vi "_29_Sample_qsns_9[5].vi"() -> ()   [LabVIEW 2020]
panel:
  out "subarray 3":i32[](array[numeric])
  out "subarray 2":i32[](array[numeric])
  out "subarray":i32[](array[numeric])
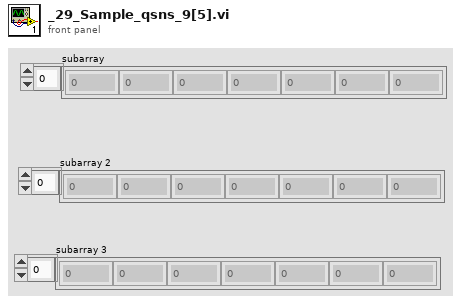
[diagram p1: front panel]
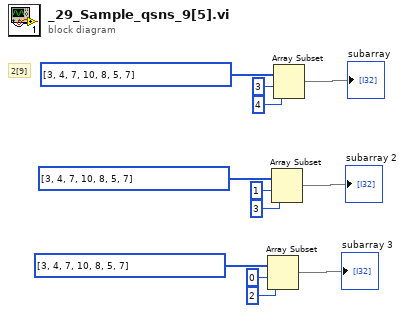
[diagram p0: block diagram]
diagram:
  # "2[9]"
  n1 = Array Subset "Array Subset"(array=i32[] [3, 4, 7, 10, 8, 5, 7], index=0, length=2) -> (→"subarray 3":i32[])
  n2 = Array Subset "Array Subset"(array=i32[] [3, 4, 7, 10, 8, 5, 7], index=1, length=3) -> (→"subarray 2":i32[])
  n3 = Array Subset "Array Subset"(array=i32[] [3, 4, 7, 10, 8, 5, 7], index=3, length=4) -> (→"subarray":i32[])
